vi "LVH5AreadI16Array.vi"(6 "error in (no error)":errorcluster, 8 "Name":string, 9 "HDF5 Location in":T1) -> (0 "error out":errorcluster, 1 "Value":i16[](array[numeric]), 3 "HDF5 Location out":T1)   [LabVIEW 2017]
doc: "This is a high level VI for writing string attributes only. It should not normally need to be called by users of LVHDF5. They should instead call Simple H5Awrite. This was implemented to break a recursion cycle in Type Caching."
uses:
  <vilib>/UPVI/lvhdf5/library.llb/HDF5 Ref.ctl
  <vilib>/UPVI/lvhdf5/datatype.llb/LVH5ClassID.ctl
  <vilib>/UPVI/lvhdf5/h5helper.dll
panel:
  # "LVHDF5 Toolkit\nCopyright (c) 2005-2013 by Jason D. Sommerville\nCopyright (c) 2014 by UPVI, LLC.\n\nThis use and distribution of this file is governed by the terms found in \nLICENSE.txt distributed with this toolkit and installed at\n <user.lib>\\_lvhdf5\\LICENSE.txt"
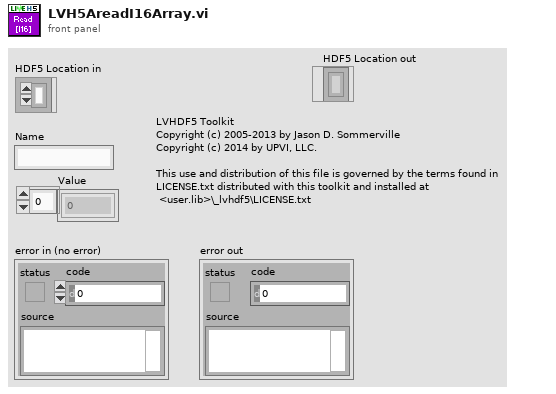
[diagram p1: front panel]
types:
  T1 = typedef "HDF5 Ref.ctl" = refnum<k1>
  T2 = typedef "LVH5ClassID.ctl" = enum32{"H5T_IEEE_F32BE", "H5T_IEEE_F32LE", "H5T_IEEE_F64BE", "H5T_IEEE_F64LE", "H5T_STD_I8BE", "H5T_STD_I8LE", "H5T_STD_I16BE", "H5T_STD_I16LE", "H5T_STD_I32BE", "H5T_STD_I32LE", "H5T_STD_I64BE", "H5T_STD_I64LE", "H5T_STD_U8BE", "H5T_STD_U8LE", "H5T_STD_U16BE", "H5T_STD_U16LE", "H5T_STD_U32BE", "H5T_STD_U32LE", "H5T_STD_U64BE", "H5T_STD_U64LE", "H5T_STD_B8BE", "H5T_STD_B8LE", "H5T_STD_B16BE", "H5T_STD_B16LE", "H5T_STD_B32BE", "H5T_STD_B32LE", "H5T_STD_B64BE", "H5T_STD_B64LE", "H5T_STD_REF_OBJ", "H5T_STD_REF_DSETREG", "H5T_UNIX_D32BE", "H5T_UNIX_D32LE", "H5T_UNIX_D64BE", "H5T_UNIX_D64LE", "H5T_C_S1", "H5T_FORTRAN_S1", "H5T_INTEL_I8", "H5T_INTEL_I16", "H5T_INTEL_I32", "H5T_INTEL_I64", "H5T_INTEL_U8", "H5T_INTEL_U16", "H5T_INTEL_U32", "H5T_INTEL_U64", "H5T_INTEL_B8", "H5T_INTEL_B16", "H5T_INTEL_B32", "H5T_INTEL_B64", "H5T_INTEL_F32", "H5T_INTEL_F64", "H5T_ALPHA_I8", "H5T_ALPHA_I16", "H5T_ALPHA_I32", "H5T_ALPHA_I64", "H5T_ALPHA_U8", "H5T_ALPHA_U16", "H5T_ALPHA_U32", "H5T_ALPHA_U64", "H5T_ALPHA_B8", "H5T_ALPHA_B16", "H5T_ALPHA_B32", "H5T_ALPHA_B64", "H5T_ALPHA_F32", "H5T_ALPHA_F64", "H5T_MIPS_I8", "H5T_MIPS_I16", "H5T_MIPS_I32", "H5T_MIPS_I64", "H5T_MIPS_U8", "H5T_MIPS_U16", "H5T_MIPS_U32", "H5T_MIPS_U64", "H5T_MIPS_B8", "H5T_MIPS_B16", "H5T_MIPS_B32", "H5T_MIPS_B64", "H5T_MIPS_F32", "H5T_MIPS_F64", "H5T_NATIVE_CHAR", "H5T_NATIVE_SCHAR", "H5T_NATIVE_UCHAR", "H5T_NATIVE_SHORT", "H5T_NATIVE_USHORT", "H5T_NATIVE_INT", "H5T_NATIVE_UINT", "H5T_NATIVE_LONG", "H5T_NATIVE_ULONG", "H5T_NATIVE_LLONG", "H5T_NATIVE_ULLONG", "H5T_NATIVE_FLOAT", "H5T_NATIVE_DOUBLE", "H5T_NATIVE_LDOUBLE", "H5T_NATIVE_B8", "H5T_NATIVE_B16", "H5T_NATIVE_B32", "H5T_NATIVE_B64", "H5T_NATIVE_OPAQUE", "H5T_NATIVE_HADDR", "H5T_NATIVE_HSIZE", "H5T_NATIVE_HSSIZE", "H5T_NATIVE_HERR", "H5T_NATIVE_HBOOL", "H5T_NATIVE_INT8", "H5T_NATIVE_UINT8", "H5T_NATIVE_INT_LEAST8", "H5T_NATIVE_UINT_LEAST8", "H5T_NATIVE_INT_FAST8", "H5T_NATIVE_UINT_FAST8", "H5T_NATIVE_INT16", "H5T_NATIVE_UINT16", "H5T_NATIVE_INT_LEAST16", "H5T_NATIVE_UINT_LEAST16", "H5T_NATIVE_INT_FAST16", "H5T_NATIVE_UINT_FAST16", "H5T_NATIVE_INT32", "H5T_NATIVE_UINT32", "H5T_NATIVE_INT_LEAST32", "H5T_NATIVE_UINT_LEAST32", "H5T_NATIVE_INT_FAST32", "H5T_NATIVE_UINT_FAST32", "H5T_NATIVE_INT64", "H5T_NATIVE_UINT64", "H5T_NATIVE_INT_LEAST64", "H5T_NATIVE_UINT_LEAST64", "H5T_NATIVE_INT_FAST64"}
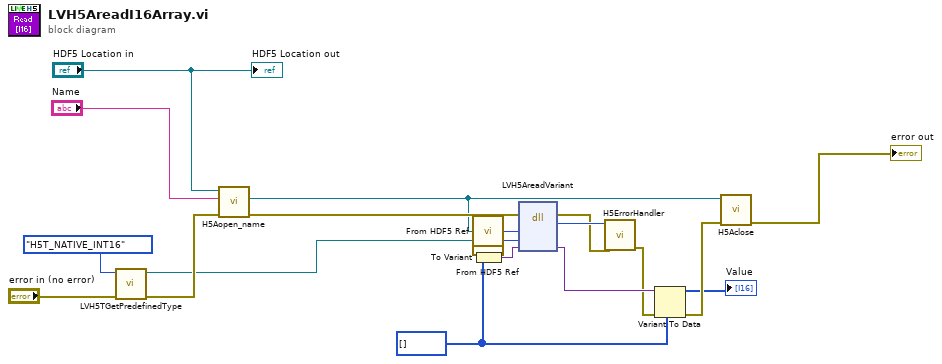
[diagram p0: block diagram]
diagram:
  w5 = i16[] [] ("Value")
  n1 = call <vilib>:"LVH5TGetPredefinedType.vi"("error in"="error in (no error)", "H5 Standard Type"=LVH5ClassID."H5T_NATIVE_INT16") -> ("error out"=w12:errorcluster, "HDF5 Ref"=w9:T1)  [unwired: 8 in]
  n2 = call <vilib>:"H5Aopen_name.vi"("error in (no error)"=w12, "name"="Name", "HDF5 Ref"="HDF5 Location in") -> ("error out"=w10:errorcluster, "HDF5 Attr Ref"=w8:T1)  [unwired: 4 in, 1 out]
  n3 = call <vilib>:"From HDF5 Ref.vi"("HDF5 Ref"=w8) -> ("I32"=w19:i32)
  n4 = call <vilib>:"From HDF5 Ref.vi"("HDF5 Ref"=w9) -> ("I32"=w11:i32)
  n5 = To Variant(anything=w5) -> (Variant=w7:variant)
  n6 = dll-call lib="C:/Program Files/National Instruments/LabVIEW 2017/vi.lib/UPVI/lvhdf5/h5helper.dll" fn="LVH5AreadVariant"(error in=w10, "attr_id"=w19, "mem_type_id"=w11, "data"=w7) -> (error out=w13:errorcluster, "return type"=w14:i32, "data"=w6:variant)  [unwired: 4 in, 1 out]
  n7 = call <vilib>:"H5ErrorHandler.vi"("error in (no error)"=w13, "herr_t"=w14) -> ("error out"=w4:errorcluster)  [unwired: 3 in, 4 out]
  n8 = Variant To Data(error in=w4, type=w5, Variant=w6) -> (data=→"Value":i16[], error out=w3:errorcluster)
  n9 = call <vilib>:"H5Aclose.vi"("error in (no error)"=w3, "HDF5 Dataset Ref"=w8) -> ("error out"=→"error out":errorcluster)  [unwired: 7 in]
  "HDF5 Location out" <- "HDF5 Location in"
